vi "get measurements.vi"(8 "error in (no error)":errorcluster, 10 "measurements":T1, 11 "id":i32) -> (0 "error out":errorcluster, 2 "measurements out":T1, 3 "function return":i32)   [LabVIEW 2012, in "libximc.lvlib"]
doc: "result_t XIMC_API get_measurements (device_t id, measurements_t* measurements);"
uses:
  libximc.lvlib
  libximc.dll
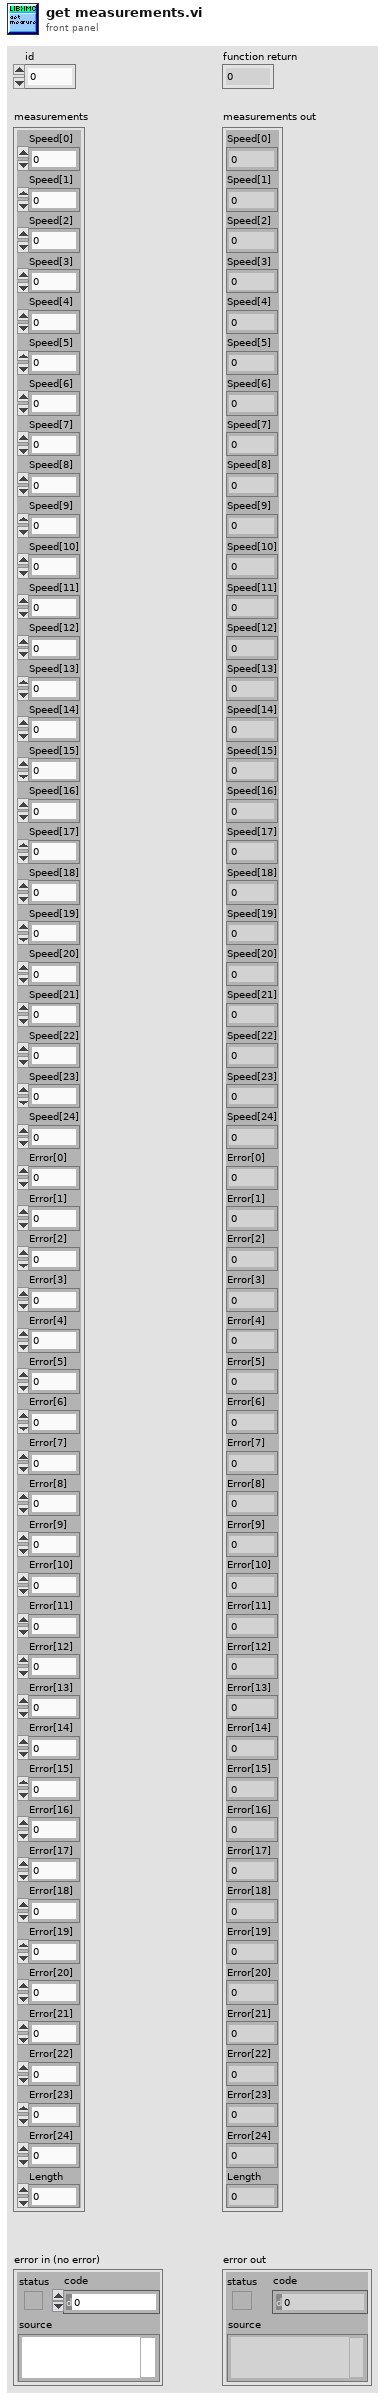
[diagram p1: front panel]
types:
  T1 = cluster{"Speed[0]":i32, "Speed[1]":i32, "Speed[2]":i32, "Speed[3]":i32, "Speed[4]":i32, "Speed[5]":i32, "Speed[6]":i32, "Speed[7]":i32, "Speed[8]":i32, "Speed[9]":i32, "Speed[10]":i32, "Speed[11]":i32, "Speed[12]":i32, "Speed[13]":i32, "Speed[14]":i32, "Speed[15]":i32, "Speed[16]":i32, "Speed[17]":i32, "Speed[18]":i32, "Speed[19]":i32, "Speed[20]":i32, "Speed[21]":i32, "Speed[22]":i32, "Speed[23]":i32, "Speed[24]":i32, "Error[0]":i32, "Error[1]":i32, "Error[2]":i32, "Error[3]":i32, "Error[4]":i32, "Error[5]":i32, "Error[6]":i32, "Error[7]":i32, "Error[8]":i32, "Error[9]":i32, "Error[10]":i32, "Error[11]":i32, "Error[12]":i32, "Error[13]":i32, "Error[14]":i32, "Error[15]":i32, "Error[16]":i32, "Error[17]":i32, "Error[18]":i32, "Error[19]":i32, "Error[20]":i32, "Error[21]":i32, "Error[22]":i32, "Error[23]":i32, "Error[24]":i32, "Length":u32}
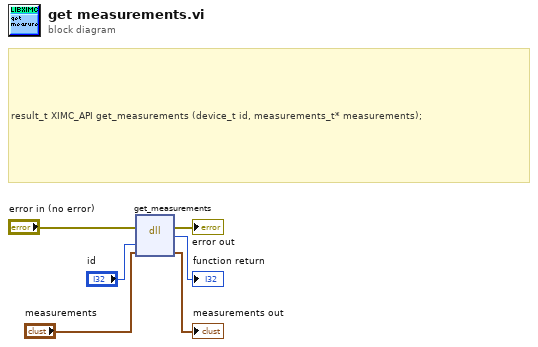
[diagram p0: block diagram]
diagram:
  # "result_t XIMC_API get_measurements (device_t id, measurements_t* measurements);"
  n1 = dll-call lib="C:/Users/Vasily/Att_examples/LabVIEW_example/libximc.*" fn="get_measurements"(error in="error in (no error)", "id"="id", "measurements"="measurements") -> (error out=→"error out":errorcluster, →"function return":i32, "measurements"=→"measurements out":T1)  [unwired: 3 in, 1 out]
